vi "FlatToRichGreeter_req.vi"(5 "OutputClusterType":T1, 11 "InputCluster":T2) -> (3 "OutputCluster":T1)   [LabVIEW 2019, in "Generated_server.lvlib"]
uses:
  Generated_server.lvlib
  Greeter_req_Flat.ctl
  Greeter_req.ctl
  Greeter_req_req_oneof/Greeter_req_req_oneof.lvclass
  Greeter_req_req_oneof/Greeter_req_req_oneof.lvclass/Greeter_req_req_oneof.ctl
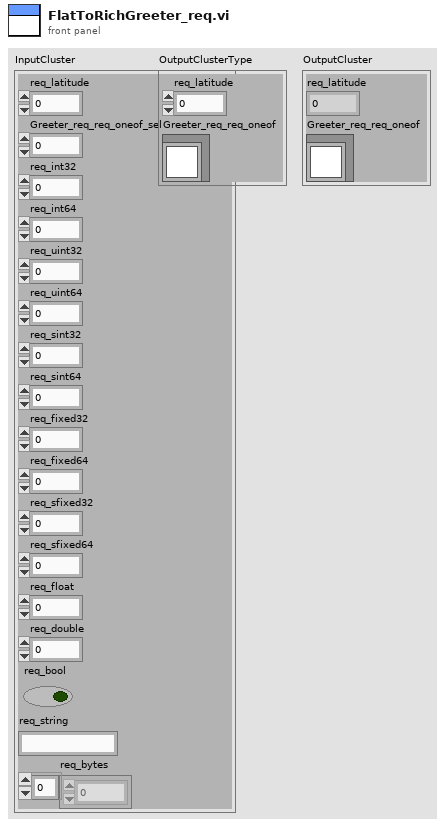
[diagram p1: front panel]
types:
  T1 = typedef "Generated_server.lvlib/Greeter_req.ctl" = cluster{"req_latitude":i32, "Greeter_req_req_oneof":refnum<class "Greeter_req_req_oneof.lvclass">}
  T2 = typedef "Generated_server.lvlib/Greeter_req_Flat.ctl" = cluster{"req_latitude":i32, "Greeter_req_req_oneof_selected_index":i32, "req_int32":i32, "req_int64":i64, "req_uint32":u32, "req_uint64":u64, "req_sint32":i32, "req_sint64":i64, "req_fixed32":u32, "req_fixed64":u64, "req_sfixed32":i32, "req_sfixed64":i64, "req_float":sgl, "req_double":dbl, "req_bool":bool, "req_string":string, "req_bytes":u8[]}
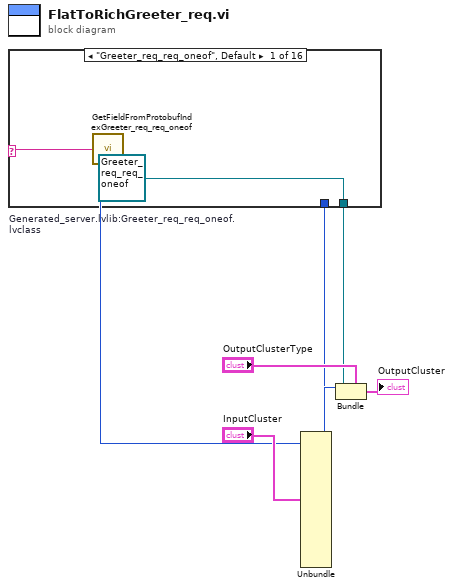
[diagram p0: block diagram]
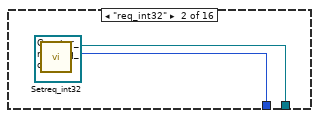
[diagram p2: hidden frame]
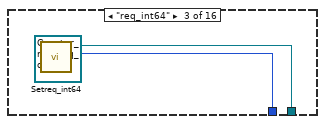
[diagram p3: hidden frame]
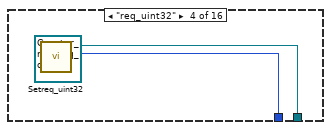
[diagram p4: hidden frame]
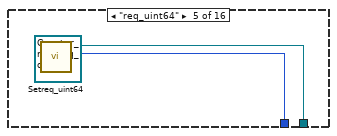
[diagram p5: hidden frame]
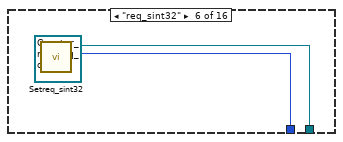
[diagram p6: hidden frame]
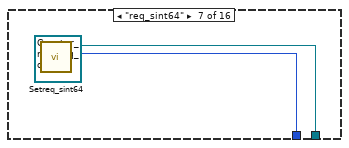
[diagram p7: hidden frame]
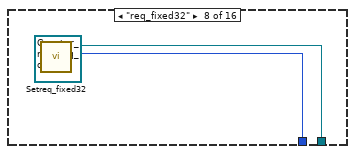
[diagram p8: hidden frame]
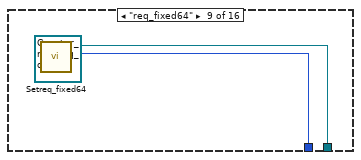
[diagram p9: hidden frame]
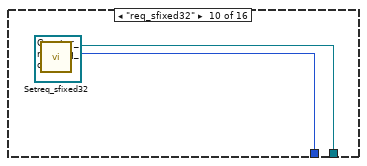
[diagram p10: hidden frame]
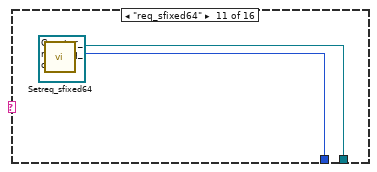
[diagram p11: hidden frame]
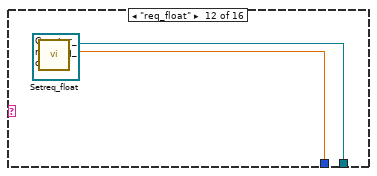
[diagram p12: hidden frame]
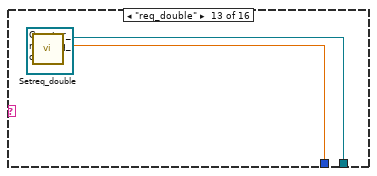
[diagram p13: hidden frame]
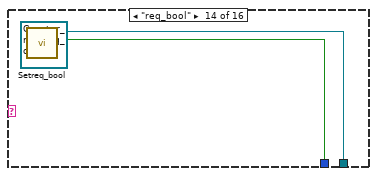
[diagram p14: hidden frame]
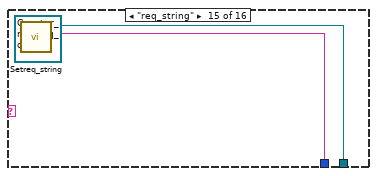
[diagram p15: hidden frame]
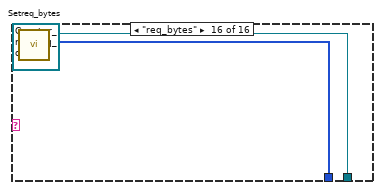
[diagram p16: hidden frame]
diagram:
  n1 = Unbundle "Unbundle"("InputCluster") -> ("req_latitude"=w19:i32, "Greeter_req_req_oneof_selected_index"=w18:i32, "req_int32"=w15:i32, "req_int64"=w14:i64, "req_uint32"=w13:u32, "req_uint64"=w12:u64, "req_sint32"=w11:i32, "req_sint64"=w10:i64, "req_fixed32"=w9:u32, "req_fixed64"=w8:u64, "req_sfixed32"=w7:i32, "req_sfixed64"=w6:i64, "req_float"=w5:sgl, "req_double"=w4:dbl, "req_bool"=w3:bool, "req_string"=w2:string, "req_bytes"=w1:u8[])
  n2 = call "GetFieldFromProtobufIndexGreeter_req_req_oneof.vi"("protobuf index"=w18) -> ("oneof field name"=w17:string)
  n3 = case "Greeter_req_req_oneof" shown="\"Greeter_req_req_oneof\", Default" w17 {
    tunnel: [w23 w25 w28 w31 w34 w37 w40 w43 w46 w49 w52 w55 w58 w61 w64 w67] -> w16
    tunnel: w15 -> [_ w26 _ _ _ _ _ _ _ _ _ _ _ _ _ _]
    tunnel: w14 -> [_ _ w29 _ _ _ _ _ _ _ _ _ _ _ _ _]
    tunnel: w13 -> [_ _ _ w32 _ _ _ _ _ _ _ _ _ _ _ _]
    tunnel: w12 -> [_ _ _ _ w35 _ _ _ _ _ _ _ _ _ _ _]
    tunnel: w11 -> [_ _ _ _ _ w38 _ _ _ _ _ _ _ _ _ _]
    tunnel: w10 -> [_ _ _ _ _ _ w41 _ _ _ _ _ _ _ _ _]
    tunnel: w9 -> [_ _ _ _ _ _ _ w44 _ _ _ _ _ _ _ _]
    tunnel: w8 -> [_ _ _ _ _ _ _ _ w47 _ _ _ _ _ _ _]
    tunnel: w7 -> [_ _ _ _ _ _ _ _ _ w50 _ _ _ _ _ _]
    tunnel: w6 -> [_ _ _ _ _ _ _ _ _ _ w53 _ _ _ _ _]
    tunnel: w5 -> [_ _ _ _ _ _ _ _ _ _ _ w56 _ _ _ _]
    tunnel: w4 -> [_ _ _ _ _ _ _ _ _ _ _ _ w59 _ _ _]
    tunnel: w3 -> [_ _ _ _ _ _ _ _ _ _ _ _ _ w62 _ _]
    tunnel: w2 -> [_ _ _ _ _ _ _ _ _ _ _ _ _ _ w65 _]
    tunnel: w1 -> [_ _ _ _ _ _ _ _ _ _ _ _ _ _ _ w68]
    frame "Greeter_req_req_oneof", Default {
      w23 = refnum<class "Greeter_req_req_oneof.lvclass"> refnum  # Generated_server.lvlib:Greeter_req_req_oneof.lvclass
    }
    frame "req_int32" {
      n4 = call "Setreq_int32.vi"("Set_Val"=w26, "OneOfTemplate in"=refnum<class "Greeter_req_req_oneof.lvclass"> refnum) -> ("OneOfTemplate out"=w25:refnum<class "Greeter_req_req_oneof.lvclass">)  [unwired: 8 in, 1 out]
    }
    frame "req_int64" {
      n5 = call "Setreq_int64.vi"("Set_Val"=w29, "OneOfTemplate in"=refnum<class "Greeter_req_req_oneof.lvclass"> refnum) -> ("OneOfTemplate out"=w28:refnum<class "Greeter_req_req_oneof.lvclass">)  [unwired: 8 in, 1 out]
    }
    frame "req_uint32" {
      n6 = call "Setreq_uint32.vi"("Set_Val"=w32, "OneOfTemplate in"=refnum<class "Greeter_req_req_oneof.lvclass"> refnum) -> ("OneOfTemplate out"=w31:refnum<class "Greeter_req_req_oneof.lvclass">)  [unwired: 8 in, 1 out]
    }
    frame "req_uint64" {
      n7 = call "Setreq_uint64.vi"("Set_Val"=w35, "OneOfTemplate in"=refnum<class "Greeter_req_req_oneof.lvclass"> refnum) -> ("OneOfTemplate out"=w34:refnum<class "Greeter_req_req_oneof.lvclass">)  [unwired: 8 in, 1 out]
    }
    frame "req_sint32" {
      n8 = call "Setreq_sint32.vi"("Set_Val"=w38, "OneOfTemplate in"=refnum<class "Greeter_req_req_oneof.lvclass"> refnum) -> ("OneOfTemplate out"=w37:refnum<class "Greeter_req_req_oneof.lvclass">)  [unwired: 8 in, 1 out]
    }
    frame "req_sint64" {
      n9 = call "Setreq_sint64.vi"("Set_Val"=w41, "OneOfTemplate in"=refnum<class "Greeter_req_req_oneof.lvclass"> refnum) -> ("OneOfTemplate out"=w40:refnum<class "Greeter_req_req_oneof.lvclass">)  [unwired: 8 in, 1 out]
    }
    frame "req_fixed32" {
      n10 = call "Setreq_fixed32.vi"("Set_Val"=w44, "OneOfTemplate in"=refnum<class "Greeter_req_req_oneof.lvclass"> refnum) -> ("OneOfTemplate out"=w43:refnum<class "Greeter_req_req_oneof.lvclass">)  [unwired: 8 in, 1 out]
    }
    frame "req_fixed64" {
      n11 = call "Setreq_fixed64.vi"("Set_Val"=w47, "OneOfTemplate in"=refnum<class "Greeter_req_req_oneof.lvclass"> refnum) -> ("OneOfTemplate out"=w46:refnum<class "Greeter_req_req_oneof.lvclass">)  [unwired: 8 in, 1 out]
    }
    frame "req_sfixed32" {
      n12 = call "Setreq_sfixed32.vi"("Set_Val"=w50, "OneOfTemplate in"=refnum<class "Greeter_req_req_oneof.lvclass"> refnum) -> ("OneOfTemplate out"=w49:refnum<class "Greeter_req_req_oneof.lvclass">)  [unwired: 8 in, 1 out]
    }
    frame "req_sfixed64" {
      n13 = call "Setreq_sfixed64.vi"("Set_Val"=w53, "OneOfTemplate in"=refnum<class "Greeter_req_req_oneof.lvclass"> refnum) -> ("OneOfTemplate out"=w52:refnum<class "Greeter_req_req_oneof.lvclass">)  [unwired: 8 in, 1 out]
    }
    frame "req_float" {
      n14 = call "Setreq_float.vi"("Set_Val"=w56, "OneOfTemplate in"=refnum<class "Greeter_req_req_oneof.lvclass"> refnum) -> ("OneOfTemplate out"=w55:refnum<class "Greeter_req_req_oneof.lvclass">)  [unwired: 8 in, 1 out]
    }
    frame "req_double" {
      n15 = call "Setreq_double.vi"("Set_Val"=w59, "OneOfTemplate in"=refnum<class "Greeter_req_req_oneof.lvclass"> refnum) -> ("OneOfTemplate out"=w58:refnum<class "Greeter_req_req_oneof.lvclass">)  [unwired: 8 in, 1 out]
    }
    frame "req_bool" {
      n16 = call "Setreq_bool.vi"("Set_Val"=w62, "OneOfTemplate in"=refnum<class "Greeter_req_req_oneof.lvclass"> refnum) -> ("OneOfTemplate out"=w61:refnum<class "Greeter_req_req_oneof.lvclass">)  [unwired: 8 in, 1 out]
    }
    frame "req_string" {
      n17 = call "Setreq_string.vi"("Set_Val"=w65, "OneOfTemplate in"=refnum<class "Greeter_req_req_oneof.lvclass"> refnum) -> ("OneOfTemplate out"=w64:refnum<class "Greeter_req_req_oneof.lvclass">)  [unwired: 8 in, 1 out]
    }
    frame "req_bytes" {
      n18 = call "Setreq_bytes.vi"("Set_Val"=w68, "OneOfTemplate in"=refnum<class "Greeter_req_req_oneof.lvclass"> refnum) -> ("OneOfTemplate out"=w67:refnum<class "Greeter_req_req_oneof.lvclass">)  [unwired: 8 in, 1 out]
    }
  }
  n19 = Bundle "Bundle"(cluster="OutputClusterType", "req_latitude"=w19, "Greeter_req_req_oneof"=w16) -> (→"OutputCluster":T1)
